vi "Configure Test Runner.vi"(8 "error in (no error)":errorcluster, 10 "Number of Test Runners":u32=1, 11 "Execution API In":refnum<class "Execution API.lvclass">) -> (0 "error out":errorcluster, 3 "Execution API Out":refnum<class "Execution API.lvclass">)   [LabVIEW 2020, in "Execution API.lvclass"]
doc: "Configure the number of test runners to launch in parallel. The configuration must be made before running the tests."
uses:
  Execution API.lvclass
  Execution API.lvclass/Execution API.ctl
  Application Framework/Process Classes/Process/Process.lvclass/Process.ctl
  Application Framework/Process Classes/Process/Protected/Messaging/Enqueue Message.vi
  Test Runner/Test Runner.lvclass
  C:/git/astemes-lunit/source/Application Framework/Process Classes/Process/Process.lvclass
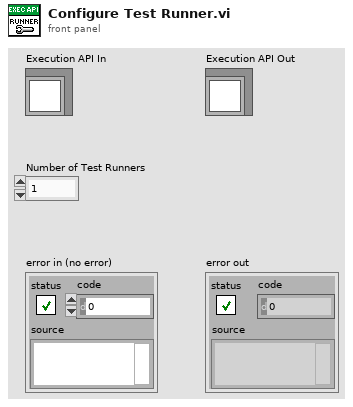
[diagram p1: front panel]
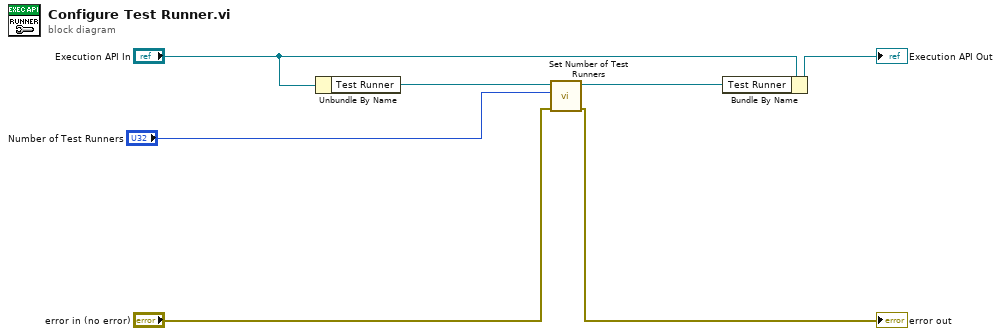
[diagram p0: block diagram]
diagram:
  n1 = Unbundle By Name("Execution API In") -> ("Test Runner"=w6:refnum<class "Test Runner.lvclass">)
  n2 = call "Set Number of Test Runners.vi"("error in (no error)"="error in (no error)", "Number of Test Runners"="Number of Test Runners", "Test Runner in"=w6) -> ("error out"=→"error out":errorcluster, "Test Runner out"=w1:refnum<class "Test Runner.lvclass">)  [unwired: 7 in]
  n3 = Bundle By Name(cluster="Execution API In", "Test Runner"=w1) -> (→"Execution API Out":refnum<class "Execution API.lvclass">)
